vi "Get Timestamp String.vi"() -> (3 "date/time string":string)   [LabVIEW 2023]
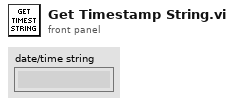
[diagram p1: front panel]
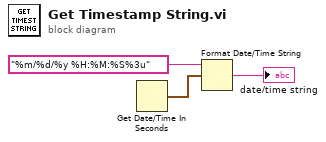
[diagram p0: block diagram]
diagram:
  n1 = Get Date/Time In Seconds() -> (seconds since 1Jan1904=w1:timestamp)
  n2 = Format Date/Time String(time format string (%c)="%m/%d/%y %H:%M:%S%3u", seconds (now)=w1) -> (date/time string=→"date/time string":string)  [unwired: 1 in]
